vi "UTIL Progress Bar Create.vi"(6 "Show Progress Bar":bool, 8 "error in (no error)":errorcluster, 9 "Message":string, 10 "High":i32, 11 "Low (0)":i32) -> (0 "error out":errorcluster, 3 "reference":refnum<vi>)   [LabVIEW 2019]
doc: "10/01/2010\n\nNational Analytics (TLE)\n\nCreate a reference to a progress bar modal pop-up vi. The progress bar can be displayed or hidden. The message can be set. The low and high range of the progress bar can be set."
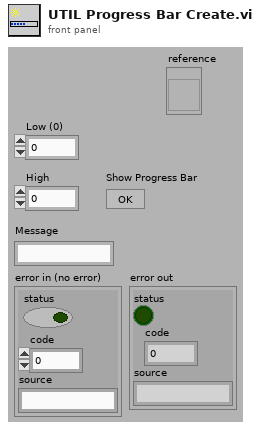
[diagram p1: front panel]
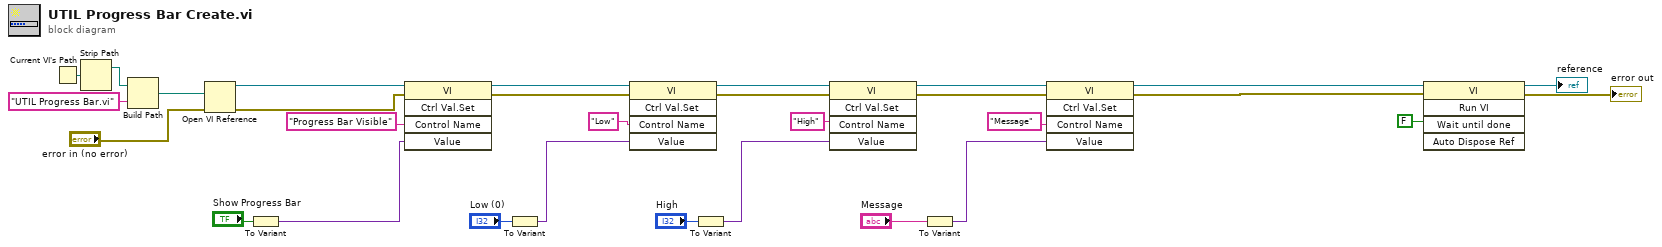
[diagram p0: block diagram]
diagram:
  n1 = Current VI's Path() -> (path=w20:path)
  n2 = Strip Path(path=w20) -> (stripped path=w21:path)  [unwired: 1 out]
  n3 = Build Path(base path=w21, name or relative path="UTIL Progress Bar.vi") -> (appended path=w23:path)
  n4 = Open VI Reference(vi path=w23, error in (no error)="error in (no error)") -> (vi reference=w3:refnum<vi>, error out=w5:errorcluster)  [unwired: 1 in, 3 out]
  n5 = To Variant(anything="Show Progress Bar") -> (Variant=w7:variant)
  n6 = invoke class="VI" method="Ctrl Val.Set"(reference=w3, error in=w5, "Control Name"="Progress Bar Visible", "Value"=w7) -> (reference out=w8:refnum<vi>, error out=w4:errorcluster)  [unwired: 1 in, 3 out]
  n7 = To Variant(anything="Low (0)") -> (Variant=w17:variant)
  n8 = invoke class="VI" method="Ctrl Val.Set"(reference=w8, error in=w4, "Control Name"="Low", "Value"=w17) -> (reference out=w28:refnum<vi>, error out=w26:errorcluster)  [unwired: 1 in, 3 out]
  n9 = To Variant(anything="High") -> (Variant=w16:variant)
  n10 = invoke class="VI" method="Ctrl Val.Set"(reference=w28, error in=w26, "Control Name"="High", "Value"=w16) -> (reference out=w13:refnum<vi>, error out=w12:errorcluster)  [unwired: 1 in, 3 out]
  n11 = To Variant(anything="Message") -> (Variant=w14:variant)
  n12 = invoke class="VI" method="Ctrl Val.Set"(reference=w13, error in=w12, "Control Name"="Message", "Value"=w14) -> (reference out=w2:refnum<vi>, error out=w1:errorcluster)  [unwired: 1 in, 3 out]
  n13 = invoke class="VI" method="Run VI"(reference=w2, error in=w1, "Wait until done"=FALSE) -> (reference out=→"reference":refnum<vi>, error out=→"error out":errorcluster)  [unwired: 2 in, 3 out]
